vi "Align Mask and Signal.vi"   [LabVIEW 2018]
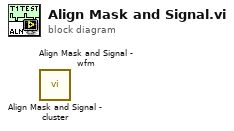
[diagram p0: block diagram]
diagram:
  n1 = call "Align Mask and Signal - cluster.vi"() -> ()  [unwired: 7 in, 5 out]
  n2 = call "Align Mask and Signal - wfm.vi"() -> ()  [unwired: 7 in, 5 out]
